vi "Database Connection.vi"(8 "error in (no error)":errorcluster) -> (0 "error out":errorcluster)   [LabVIEW 2013]
uses:
  Public API/Post_Dust_Event.ctl
  Private/Controls/File_location.ctl
  Public API/DisplayExperimentSetting.ctl
  Private/Controls/Dust_Properties.ctl
  Private/Controls/source_builders.ctl
  Private/Controls/Operator.ctl
  Private/Controls/dust_type_indicator.ctl
  Small Accelerator/Post_Dust_Event_small.ctl
  <vilib>/Utility/miscctls.llb/LVPointTypeDef.ctl
  Public API/Dust_Event.ctl
  Public API/Signal.ctl
  Private/Controls/Role ID.ctl
  Private/Controls/Hardware ID.ctl
  Private/Controls/Estimate_source.ctl
  Functional Global Variables/Action Items.ctl
  Private/UI Elements/throttle.vi
  Private/Sub-Polymorphic/post_dust_event_small.vi
  Private/Sub-Polymorphic/post_dust_event_big.vi
panel:
  in  "Tab Control":enum32{"Status", "Processing", "Error Handling"}(tab)
  out "Small?":bool
  out "Dust Properties":T1
  in  "Update dust info":bool
  in  "Update Experiment Settings":bool
  out "output cluster 2":T2={"Current Experiment Name:"="NDA", "Current Experiment Description:"="Database testing during NDA run in August.", "Current Experiment Group ID:"="Database Testing", "Experiment Settings Last Updated At:"=timestamp(3427974586.5021 s since 1904-01-01)}
  out "Dust Type":T3 {"Batch" step=1; "Type" step=1; "Dust Source Builder:" items=["Keith Drake", "Nick Beaty", "Anthony Shu", "David James", "John Fontanese"]}
  in  "Update Operator":bool
  out "Current Operator:":T5 {"Operator" items=["Giraffe", "Andrew Collette", "Keith Drake", "Anthony Shu", "Evan Thomas", "Nicholaus Beaty", "David James", "John Fontanese", ""]}
  out "# Events posted during current session:":i32=96
  out "# Events in dust event queue:":i32=388
  out "Dust Event Processing Big":T6={"Dust Event ID"=0, "Integer Timestamp"=13461087072182, "Velocity"=nan, "Mass"=nan, "Charge"=2.2111935e-15, "Radius"=0.0, "Experiment Settings"=0.0, "Pelletron ID"=0, "Estimate Quality"=0.0, "File Location"=0, "id_dust_info"=0.0} {"File Location" items=["Unknown"=-1, "Processing"=0, "Storage"=1]}
  out "Dust Event Processing Small":T8 {"File Location" items=["Unknown"=-1, "Processing"=0, "Storage"=1]}
  in  "Write Signals":bool=TRUE
  out "Test":bool caption="Test Database in use:"
  out "Test 2":bool=TRUE caption="Production Database in use:"
  in  "Clear Errors":bool
  in  "Exit":bool=TRUE
  # "Database Connection V3"
  # "Experiment Status:"
  # "Dust Information"
  # "Dust Event"
  # "Dust Event Small"
  # "ODBC Connection Status:"
  # "Error Status:"
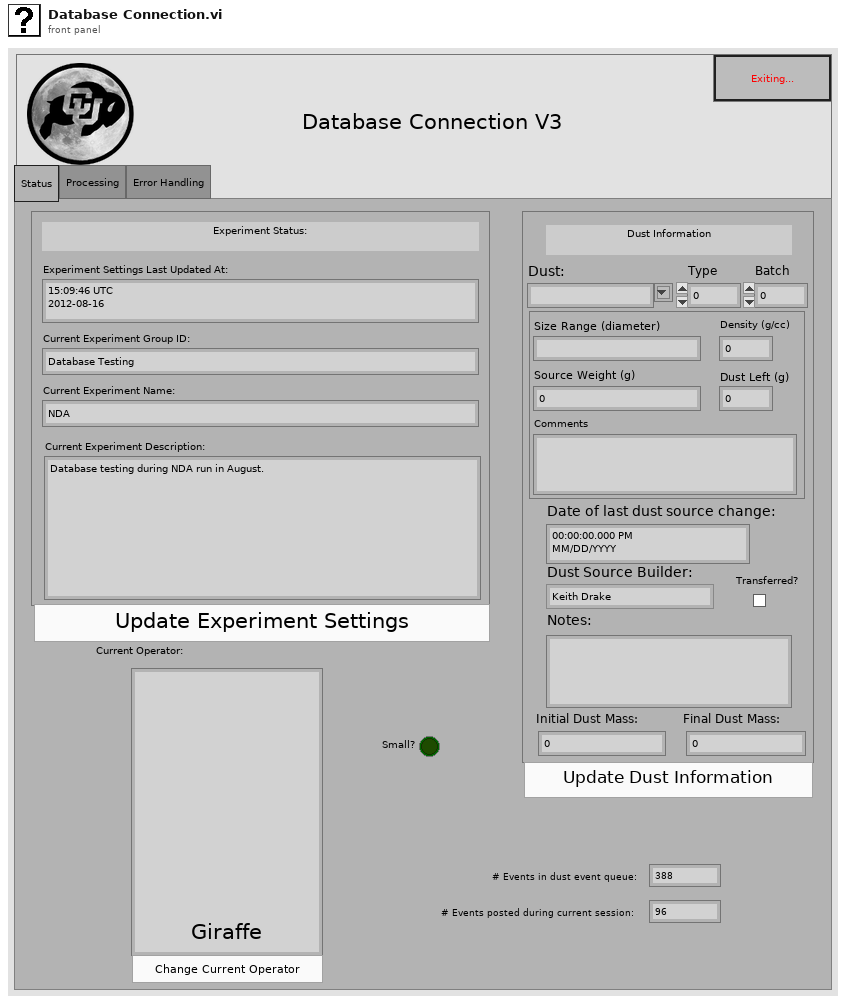
[diagram p1: front panel]
types:
  T1 = typedef "dust_type_indicator.ctl" = cluster{"id_dust_type":i32, "Size Range (diameter)":string, "Density (g/cc)":dbl, "Source Weight (g)":dbl, "Dust Left (g)":dbl, "Comments":string}
  T2 = typedef "DisplayExperimentSetting.ctl" = cluster{"Current Experiment Name:":string, "Current Experiment Description:":string, "Current Experiment Group ID:":string, "Experiment Settings Last Updated At:":timestamp}
  T3 = typedef "Dust_Properties.ctl" = cluster{"Dust info id":u16, "Integer Timestamp":i64, "Dust:":string, "Dust Source Builder:":T4, "Notes:":string, "Date of last dust source change:":timestamp, "Initial Dust Mass:":dbl, "Final Dust Mass:":dbl, "Type":u16, "Batch":u16, "dust type id":u16, "Transferred?":bool}
  T4 = typedef "source_builders.ctl" = u16
  T5 = typedef "Operator.ctl" = cluster{"Timestamp":i64, "Operator":u16}
  T6 = typedef "Post_Dust_Event.ctl" = cluster{"Dust Event ID":i64, "Integer Timestamp":i64, "Velocity":sgl, "Mass":sgl, "Charge":sgl, "Radius":sgl, "Experiment Settings":dbl, "Pelletron ID":i32, "Estimate Quality":sgl, "File Location":T7, "id_dust_info":dbl}
  T7 = typedef "File_location.ctl" = i8
  T8 = typedef "Post_Dust_Event_small.ctl" = cluster{"Dust Event ID":i64, "Integer Timestamp":i64, "Velocity":sgl, "Mass":sgl, "Charge":sgl, "Radius":sgl, "Needle Voltage (MV)":dbl, "Experiment Settings":dbl, "Estimate Quality":sgl, "File Location":T7, "id_dust_info":dbl}
  T9 = typedef "LVPointTypeDef.ctl" = cluster{"Horizontal":i16, "Vertical":i16}
  T10 = typedef "Dust_Event.ctl" = cluster{"Time Stamp":timestamp, "Velocity":sgl, "Mass":sgl, "Charge":sgl, "Radius":sgl, "Array":T11[], "Dust Event ID":i64, "Passed_3rd_Detector":bool, "Estimate Source":T14, "Estimate Quality":sgl}
  T11 = typedef "Signal.ctl" = cluster{"Signal ID":i64, "Time Stamp":timestamp, "Dust Event ID":i64, "Role ID":T12, "Data":sgl[], "Signal Length":i32, "dt":sgl, "Offset":dbl, "Hardware ID":T13}
  T12 = typedef "Role ID.ctl" = enum16{"First_Detector", "Second_Detector", "Third_Detector", "LeCroy_CH1", "LeCroy_CH2", "LeCroy_CH3", "LeCroy_CH4", "PSU", "DCS 1", "DCS 2"}
  T13 = typedef "Hardware ID.ctl" = enum16{"Unknown", "CSA 1", "CSA 2", "CSA 3", "CSA 4", "CSA 5", "CSA 6", "DCS 1", "DCS 2"}
  T14 = typedef "Estimate_source.ctl" = i8
  T15 = typedef "Action Items.ctl" = enum16{"Initialize", "Get", "Set"}
  T16 = typedef "NI_Database_API.lvlib/Conn ObjectReference.ctl" = refnum<k1>
  T17 = typedef "Semaphore RefNum" = refnum<k1>
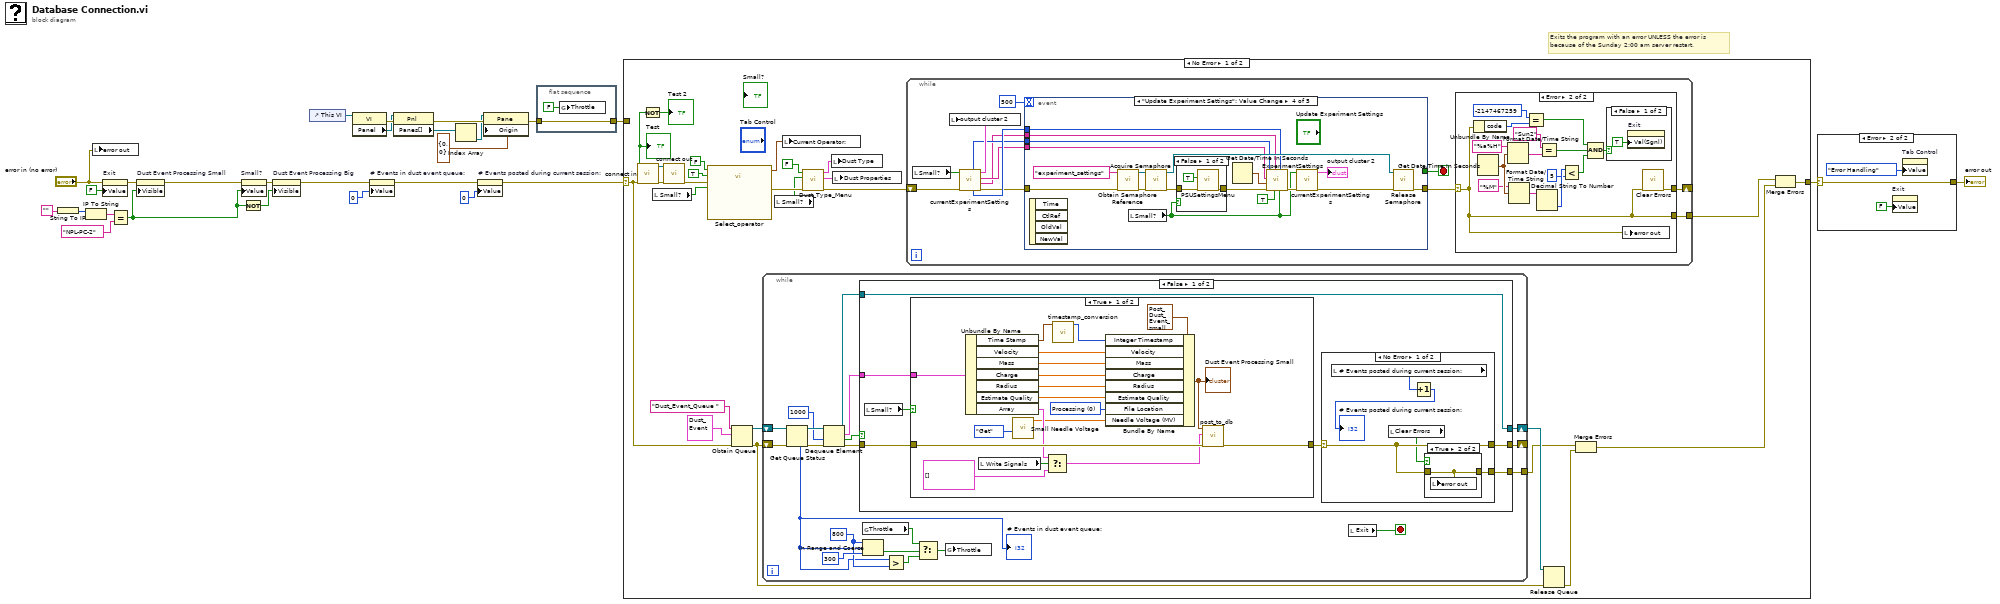
[diagram p0: block diagram]
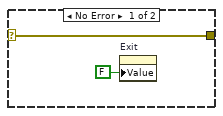
[diagram p2: hidden frame]
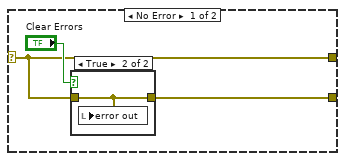
[diagram p3: hidden frame]
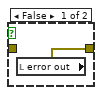
[diagram p4: hidden frame]
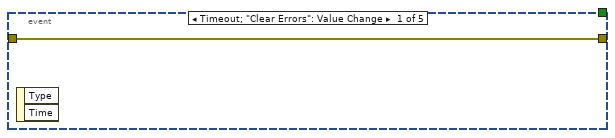
[diagram p6: hidden frame]
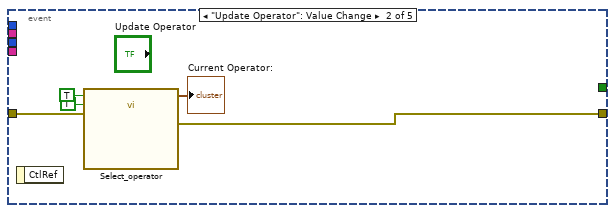
[diagram p7: hidden frame]
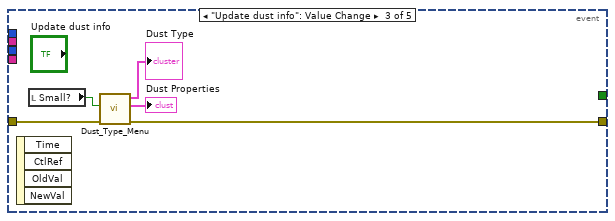
[diagram p8: hidden frame]
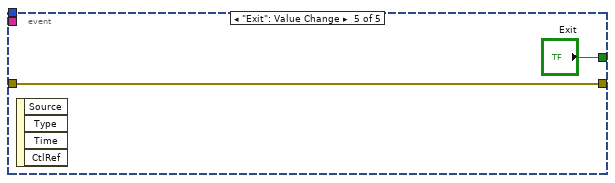
[diagram p10: hidden frame]
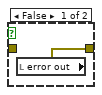
[diagram p11: hidden frame]
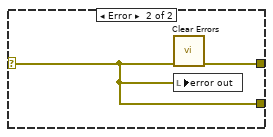
[diagram p12: hidden frame]
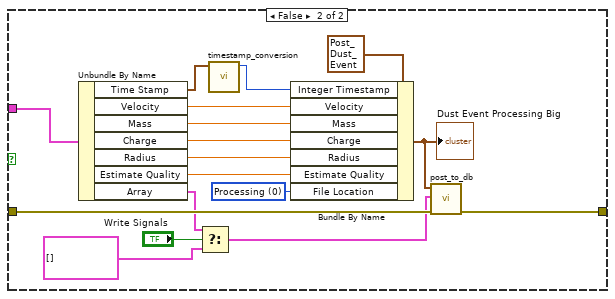
[diagram p13: hidden frame]
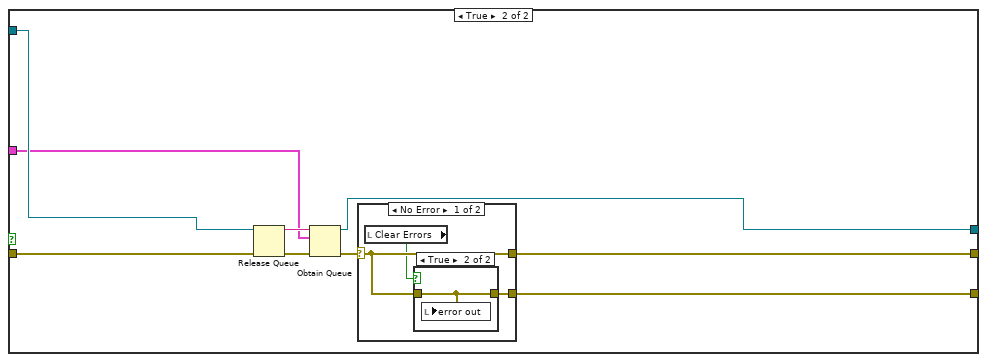
[diagram p14: hidden frame]
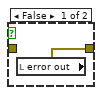
[diagram p15: hidden frame]
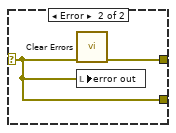
[diagram p16: hidden frame]
diagram:
  # "Exits the program with an error UNLESS the error is\nbecause of the Sunday 2:00 am server restart."
  n1 = String To IP(1:"") -> (0:w15:u32)
  n2 = IP To String(2:w15) -> (0:w14:string)  [unwired: 1 in]
  n3 = local write "error out"("error in (no error)") -> ()
  n4 = property on="Exit" class="Bool (strict)"(error in="error in (no error)", "Value"=FALSE ("Exit")) -> (error out=w20:errorcluster)  [unwired: 1 in, 1 out]
  n5 = Equal?(x=w14, y="NPL-PC-2") -> (x = y?=w10:bool)
  n6 = property on="Dust Event Processing Small" class="Clust (strict)"(error in=w20, "Visible"=w10) -> (error out=w9:errorcluster)  [unwired: 1 in, 1 out]
  n7 = property on="Small?" class="Bool (strict)"(error in=w9, "Value"=w10) -> (error out=w8:errorcluster)  [unwired: 1 in, 1 out]
  n8 = Not(x=w10) -> (.not. x?=w7:bool)
  n9 = property on="Dust Event Processing Big" class="Clust (strict)"(error in=w8, "Visible"=w7) -> (error out=w5:errorcluster)  [unwired: 1 in, 1 out]
  n10 = control-ref of="This VI"() -> (w27:refnum<vi>)
  n11 = property class="VI"(reference=w27) -> (error out=w26:errorcluster, "Panel"=w25:refnum<vi>)  [unwired: 1 in, 1 out]
  n12 = property on="# Events in dust event queue:" class="DigNum (strict)"(error in=w5, "Value"=0 ("# Events in dust event queue:")) -> (error out=w3:errorcluster)  [unwired: 1 in, 1 out]
  n13 = property class="Pnl"(reference=w25, error in=w26) -> (error out=w24:errorcluster, "Panes[]"=w23:refnum<vi>[])  [unwired: 1 out]
  n14 = Index Array(array=w23) -> (element=w22:refnum<vi>)  [unwired: 1 in]
  n15 = property on="# Events posted during current session:" class="DigNum (strict)"(error in=w3, "Value"=0 ("# Events in dust event queue:")) -> (error out=w2:errorcluster)  [unwired: 1 in, 1 out]
  n16 = property class="Pane"(reference=w22, error in=w24, "Origin"=T9 {"Horizontal"=0, "Vertical"=0}) -> (error out=w17:errorcluster)  [unwired: 1 out]
  n17 = flat-sequence {
    tunnel: [w29] -> w18
    tunnel: w17 -> [w29]
    frame #0 {
      n18 = global write "throttle.vi" "Throttle"(FALSE ("Throttle")) -> ()
    }
  }
  n19 = case shown="No Error" w2 {
    selector: w2 -> [w36 w214]
    tunnel: [w44 w214] -> w12
    tunnel: w18 -> [_ _]
    frame No Error {
      n20 = call "connect in.vi"("error in (no error)"=w36) -> ("error out"=w39:errorcluster, "Database Connection"=w40:T16, "Test Server"=w38:bool)  [unwired: 6 in]
      "Test" <- w38
      n21 = Not(x=w38) -> (.not. x?=→"Test 2":bool)
      n22 = local read "Small?"() -> (w43:bool)
      n23 = call "connect out.vi"("error in (no error)"=w39, "connection reference"=w40) -> ("error out"=w37:errorcluster)  [unwired: 9 in]
      n24 = call "Select_operator.vi"("Enable"=FALSE, "sub vi?"=TRUE, "error in (no error)"=w37, "small?"=w43) -> ("Operator Cluster 2"=w48:T5, "error out"=w35:errorcluster)  [unwired: 13 in, 1 out]
      n25 = Obtain Queue(name (unnamed)="Dust_Event_Queue ", element data type=T10 {"Time Stamp"=timestamp(0 s since 1904-01-01), "Velocity"=0.0, "Mass"=0.0, "Charge"=0.0, "Radius"=0.0, "Array"=[], "Dust Event ID"=0, "Passed_3rd_Detector"=FALSE, "Estimate Source"=0, "Estimate Quality"=0.0} ("Cluster"), error in (no error)=w36) -> (queue out=w52:refnum<queue>, error out=w54:errorcluster)  [unwired: 2 in, 1 out]
      n26 = while {
        shift-right: [w129] -> _
        shift-left: w54 -> [w144]
        shift-right: [w143] -> w53
        shift-left: w52 -> [w145]
        tunnel: [w127] -> w41
        stop <- w128 stop-if-true
        w134 = 800 ("y")
        n27 = Get Queue Status(queue=w145, error in (no error)=w144) -> (queue out=w141:refnum<queue>, error out=w139:errorcluster, # elements in queue=w126:i32)  [unwired: 1 in, 5 out]
        "# Events in dust event queue:" <- w126
        n28 = Dequeue Element(queue=w141, timeout in ms (-1)=u32 1000 ("milliseconds to wait"), error in (no error)=w139) -> (queue out=w140:refnum<queue>, element=w142:T10, timed out?=w137:bool, error out=w138:errorcluster)
        n29 = case shown="False" w137 {
          tunnel: w140 -> [w152 w206]
          tunnel: w138 -> [w150 w198]
          tunnel: [w152 w204] -> w143
          tunnel: [w147 w200] -> w129
          tunnel: w142 -> [w151 w202]
          tunnel: [w146 w199] -> w127
          frame False {
            n30 = local read "Small?"() -> (w149:bool)
            n31 = case shown="True" w149 {
              tunnel: w151 -> [w172 w189]
              tunnel: w150 -> [w171 w188]
              tunnel: [w170 w187] -> w148
              frame True {
                w167 = T7 0 items=["Unknown"=-1, "Processing"=0, "Storage"=1] ("File Location")
                n32 = Unbundle By Name(w172) -> ("Time Stamp"=w179:timestamp, "Velocity"=w175:sgl, "Mass"=w176:sgl, "Charge"=w177:sgl, "Radius"=w178:sgl, "Estimate Quality"=w166:sgl, "Array"=w165:T11[])
                n33 = local read "Write Signals"() -> (w164:bool)
                n34 = call "Small Needle Voltage.vi"("Action"=Action_Items."Get") -> ("Output Pelletron Voltage"=w162:dbl)  [unwired: 10 in]
                n35 = Select(t=w165, s=w164, f=T11[] []) -> (s? t:f=w168:T11[])
                n36 = call "timestamp_conversion.vi"("Time Stamp"=w179) -> ("Integer Time"=w180:i64)  [unwired: 8 in, 1 out]
                n37 = Bundle By Name(cluster=T8 {"Dust Event ID"=0, "Integer Timestamp"=0, "Velocity"=0.0, "Mass"=0.0, "Charge"=0.0, "Radius"=0.0, "Needle Voltage (MV)"=0.0, "Experiment Settings"=0.0, "Estimate Quality"=0.0, "File Location"=0, "id_dust_info"=0.0} ("Cluster"), "Integer Timestamp"=w180, "Velocity"=w175, "Mass"=w176, "Charge"=w177, "Radius"=w178, "Estimate Quality"=w166, "File Location"=w167, "Needle Voltage (MV)"=w162) -> (w173:T8)
                "Dust Event Processing Small" <- w173
                n38 = call-poly "post_to_db.vi"("error in (no error)"=w171, "Signal Array"=w168, "Cluster"=w173) -> ("error out"=w170:errorcluster)  [unwired: 5 in, 3 out]
              }
              frame False {
                w183 = T7 0 items=["Unknown"=-1, "Processing"=0, "Storage"=1] ("File Location")
                n39 = Unbundle By Name(w189) -> ("Time Stamp"=w196:timestamp, "Velocity"=w192:sgl, "Mass"=w193:sgl, "Charge"=w194:sgl, "Radius"=w195:sgl, "Estimate Quality"=w182:sgl, "Array"=w181:T11[])
                n40 = Select(t=w181, s="Write Signals", f=T11[] []) -> (s? t:f=w184:T11[])
                n41 = call "timestamp_conversion.vi"("Time Stamp"=w196) -> ("Integer Time"=w197:i64)  [unwired: 8 in, 1 out]
                n42 = Bundle By Name(cluster=T6 {"Dust Event ID"=0, "Integer Timestamp"=0, "Velocity"=0.0, "Mass"=0.0, "Charge"=0.0, "Radius"=0.0, "Experiment Settings"=0.0, "Pelletron ID"=0, "Estimate Quality"=0.0, "File Location"=0, "id_dust_info"=0.0} ("Cluster 2"), "Integer Timestamp"=w197, "Velocity"=w192, "Mass"=w193, "Charge"=w194, "Radius"=w195, "Estimate Quality"=w182, "File Location"=w183) -> (w190:T6)
                "Dust Event Processing Big" <- w190
                n43 = call-poly "post_to_db.vi"("error in (no error)"=w188, "Signal Array"=w184, "Cluster"=w190) -> ("error out"=w187:errorcluster)  [unwired: 5 in, 3 out]
              }
            }
            n44 = case shown="No Error" w148 {
              selector: w148 -> [w157 w160]
              tunnel: [w157 w161] -> w147
              tunnel: [w156 w160] -> w146
              frame No Error {
                n45 = local read "# Events posted during current session:"() -> (w154:i32)
                n46 = local read "Clear Errors"() -> (w155:bool)
                n47 = Increment(x=w154) -> (x+1=→"# Events posted during current session:":i32)
                n48 = case shown="True" w155 {
                  tunnel: w157 -> [_ w159]
                  tunnel: [w158 w159] -> w156
                  frame False {
                    n49 = local read "error out"() -> (w158:errorcluster)
                  }
                  frame True {
                    n50 = local write "error out"(w159) -> ()
                  }
                }
              }
              frame Error {
                n51 = call <vilib>:"Clear Errors.vi"("error in (no error)"=w160) -> ("error out"=w161:errorcluster)  [unwired: 6 in]
                n52 = local write "error out"(w160) -> ()
              }
            }
          }
          frame True {
            n53 = Release Queue(queue=w206, error in (no error)=w198) -> (queue name=w203:string, error out=w205:errorcluster)  [unwired: 1 in, 1 out]
            n54 = Obtain Queue(name (unnamed)=w203, element data type=w202, error in (no error)=w205) -> (queue out=w204:refnum<queue>, error out=w201:errorcluster)  [unwired: 2 in, 1 out]
            n55 = case shown="No Error" w201 {
              selector: w201 -> [w209 w212]
              tunnel: [w209 w213] -> w200
              tunnel: [w208 w212] -> w199
              frame No Error {
                n56 = local read "Clear Errors"() -> (w207:bool)
                n57 = case shown="True" w207 {
                  tunnel: w209 -> [_ w211]
                  tunnel: [w210 w211] -> w208
                  frame False {
                    n58 = local read "error out"() -> (w210:errorcluster)
                  }
                  frame True {
                    n59 = local write "error out"(w211) -> ()
                  }
                }
              }
              frame Error {
                n60 = call <vilib>:"Clear Errors.vi"("error in (no error)"=w212) -> ("error out"=w213:errorcluster)  [unwired: 6 in]
                n61 = local write "error out"(w212) -> ()
              }
            }
          }
        }
        n62 = global read "throttle.vi" "Throttle"() -> (w130:bool)
        n63 = In Range and Coerce(upper limit=w134, x=w126, lower limit=300) -> (In Range?=w133:bool)  [unwired: 1 out]
        n64 = Greater?(x=w126, y=w134) -> (0:w132:bool)
        n65 = Select(t=w130, s=w133, f=w132) -> (s? t:f=w131:bool)
        n66 = global write "throttle.vi" "Throttle"(w131) -> ()
        n67 = local read "Exit"() -> (w128:bool)
      }
      n68 = local read "Small?"() -> (w31:bool)
      n69 = local write "Current Operator:"(w48) -> ()
      n70 = call "Dust_Type_Menu.vi"("error in (no error)"=w35, "Small?"=w31, "Enable"=FALSE) -> ("error out"=w34:errorcluster, "Dust Properties"=w32:T1, "Dust Info"=w33:T3)  [unwired: 5 in, 1 out]
      n71 = local write "Dust Type"(w33) -> ()
      n72 = local write "Dust Properties"(w32) -> ()
      n73 = while {
        shift-right: [w57] -> _
        shift-left: w34 -> [w67]
        tunnel: [w56] -> w42
        stop <- w59 stop-if-true
        n74 = local read "Small?"() -> (w60:bool)
        n75 = call "currentExperimentSettings.vi"("error in (no error)"=w67, "small?"=w60) -> ("error out"=w64:errorcluster, "Last Name"=w61:string, "Last Description"=w62:string, "output cluster"=w65:T2, "Experiment ID"=w66:u64, "Group ID"=w63:u64)  [unwired: 4 in]
        n76 = local write "output cluster 2"(w65) -> ()
        n77 = event shown="[3] \"Update Experiment Settings\": Value Change" {
          selector: _ -> [_ _ _ _ _]
          dyn-events: _ -> [_ _ _ _ _]
          timeout: 500 -> [_ _ _ _ _]
          tunnel: w64 -> [w91 w96 w99 w113 w124]
          tunnel: [w91 w93 w100 w112 w124] -> w58
          tunnel: w66 -> [_ _ _ w111 _]
          tunnel: w63 -> [_ _ _ w105 _]
          tunnel: w62 -> [_ _ _ w104 _]
          tunnel: w61 -> [_ _ _ w103 _]
          tunnel: [_ _ _ _ "Exit"] -> w59
          event Timeout; "Clear Errors": Value Change {
            n78 = event-data() -> ()  [unwired: 1 in, 2 out]
          }
          event "Update Operator": Value Change {
            n79 = event-data() -> ()  [unwired: 1 in, 1 out]
            n80 = call "Select_operator.vi"("Enable"=TRUE, "sub vi?"=TRUE, "error in (no error)"=w96) -> ("Operator Cluster 2"=→"Current Operator:":T5, "error out"=w93:errorcluster)  [unwired: 14 in, 1 out]
          }
          event "Update dust info": Value Change {
            n81 = event-data() -> ()  [unwired: 1 in, 4 out]
            n82 = local read "Small?"() -> (w97:bool)
            n83 = call "Dust_Type_Menu.vi"("error in (no error)"=w99, "Small?"=w97) -> ("error out"=w100:errorcluster, "Dust Properties"=→"Dust Properties":T1, "Dust Info"=→"Dust Type":T3)  [unwired: 6 in, 1 out]
          }
          event "Update Experiment Settings": Value Change {
            n84 = event-data() -> ()  [unwired: 1 in, 4 out]
            n85 = call <vilib>:"Obtain Semaphore Reference.vi"("error in (no error)"=w113, "name (unnamed)"="experiment_settings") -> ("error out"=w116:errorcluster, "semaphore"=w117:T17)  [unwired: 3 in, 1 out]
            n86 = local read "Small?"() -> (w102:bool)
            n87 = call <vilib>:"Acquire Semaphore.vi"("error in (no error)"=w116, "semaphore"=w117) -> ("error out"=w107:errorcluster, "semaphore out"=w114:T17)  [unwired: 3 in, 1 out]
            n88 = case shown="False" w102 {
              tunnel: w107 -> [w122 w123]
              tunnel: [w120 w123] -> w106
              frame False {
                n89 = call "PSUSettingsMenu.vi"("error in (no error)"=w122, "sub vi?"=TRUE) -> ("error out"=w120:errorcluster)  [unwired: 7 in, 2 out]
              }
              frame True {
              }
            }
            n90 = Get Date/Time In Seconds() -> (seconds since 1Jan1904=w119:timestamp)
            n91 = call "ExperimentSettings.vi"("small?"=w102, "Experiment Settings id"=w111, "Enable"=TRUE, "Default Experiment Name"=w103, "error in (no error)"=w106, "current time"=w119, "default Experiment Description"=w104, "Default Group ID"=w105) -> ("error out"=w110:errorcluster)  [unwired: 2 in, 1 out]
            n92 = call "currentExperimentSettings.vi"("error in (no error)"=w110, "small?"=w102) -> ("error out"=w108:errorcluster, "output cluster"=→"output cluster 2":T2)  [unwired: 4 in, 4 out]
            n93 = call <vilib>:"Release Semaphore.vi"("error in (no error)"=w108, "semaphore"=w114) -> ("error out"=w112:errorcluster)  [unwired: 4 in, 1 out]
          }
          event "Exit": Value Change {
            n94 = event-data() -> ()  [unwired: 1 in, 4 out]
          }
        }
        n95 = case shown="Error" w58 {
          selector: w58 -> [w70 w85]
          tunnel: [w70 w89] -> w57
          tunnel: [w69 w85] -> w56
          frame No Error {
            n96 = case shown="True" "Clear Errors" {
              tunnel: w70 -> [_ w73]
              tunnel: [w72 w73] -> w69
              frame False {
                n97 = local read "error out"() -> (w72:errorcluster)
              }
              frame True {
                n98 = local write "error out"(w73) -> ()
              }
            }
          }
          frame Error {
            n99 = Unbundle By Name(w85) -> ("code"=w87:i32)
            n100 = Get Date/Time In Seconds() -> (seconds since 1Jan1904=w82:timestamp)
            n101 = Format Date/Time String(time format string (%c)="%a%H", seconds (now)=w82) -> (date/time string=w83:string)  [unwired: 1 in]
            n102 = Format Date/Time String(time format string (%c)="%M", seconds (now)=w82) -> (date/time string=w80:string)  [unwired: 1 in]
            n103 = Equal?(x=-2147467259 ("y"), y=w87) -> (x = y?=w77:bool)
            n104 = Decimal String To Number(string=w80) -> (number=w79:i32)  [unwired: 2 in, 1 out]
            n105 = Equal?(x="Sun2", y=w83) -> (x = y?=w76:bool)
            n106 = Less?(x=w79, y=5) -> (x < y?=w75:bool)
            n107 = Compound Arithmetic op=AND(w77, w76, w75) -> (w74:bool)
            n108 = case shown="False" w74 {
              frame False {
                n109 = property on="Exit" class="Bool (strict)"("Val(Sgnl)"=TRUE ("Value (Signaling)")) -> ()  [unwired: 2 in, 2 out]
              }
              frame True {
              }
            }
            n110 = local write "error out"(w85) -> ()
            n111 = call <vilib>:"Clear Errors.vi"("error in (no error)"=w85) -> ("error out"=w89:errorcluster)  [unwired: 6 in]
          }
        }
      }
      n112 = Release Queue(queue=w53, error in (no error)=w54) -> (error out=w45:errorcluster)  [unwired: 1 in, 2 out]
      n113 = Merge Errors(w41, w45) -> (w46:errorcluster)
      n114 = Merge Errors(w42, w46) -> (w44:errorcluster)
    }
    frame Error {
    }
  }
  n115 = case shown="Error" w12 {
    selector: w12 -> [w216 w219]
    tunnel: [w216 w219] -> w11
    frame No Error {
      n116 = property on="Exit" class="Bool (strict)"("Value"=FALSE ("Exit")) -> ()  [unwired: 2 in, 2 out]
    }
    frame Error {
      n117 = property on="Exit" class="Bool (strict)"("Value"=FALSE ("Exit")) -> ()  [unwired: 2 in, 2 out]
      n118 = property on="Tab Control" class="TabCtl (strict)"("Value"=enum32{"Status", "Processing", "Error Handling"}."Error Handling" ("Tab Control")) -> ()  [unwired: 2 in, 2 out]
    }
  }
  "error out" <- w11
